vi "CTC_Test.vi"() -> ()   [LabVIEW 2011]
panel:
  out "Ain15":dbl format="%.3f"
  out "Ain14":dbl format="%.3f"
  out "Ain13":dbl format="%.3f"
  out "Ain12":dbl format="%.3f"
  out "Ain11":dbl format="%.3f"
  out "Ain10":dbl format="%.3f"
  out "Ain9":dbl format="%.3f"
  out "Ain8":dbl format="%.3f"
  out "Input err":string
  out "Din32":bool
  out "Din31":bool
  out "Din30":bool
  out "Din29":bool
  out "Din28":bool
  out "Din27":bool
  out "Din26":bool
  out "Din25":bool
  out "Din24":bool
  out "Din23":bool
  out "Din22":bool
  out "Din21":bool
  out "Din20":bool
  out "Din19":bool
  out "Din18":bool
  out "Din17":bool
  out "Din16":bool
  out "Din15":bool
  out "Din14":bool
  out "Din13":bool
  out "Din12":bool
  out "Din11":bool
  out "Din10":bool
  out "Din9":bool
  out "Din8":bool
  out "Din7":bool
  out "Din6":bool
  out "Din5":bool
  out "Din4":bool
  out "Din3":bool
  out "Din2":bool
  out "Din1":bool
  in  "Din Board":u8=1 min=1
  in  "Dout Board":u8=1 min=1
  out "Ain7":dbl format="%.3f"
  in  "Aout8":dbl min=0.0 max=2000.0 format="%.1f"
  out "Ain6":dbl format="%.3f"
  in  "Aout7":dbl min=0.0 max=2000.0 format="%.1f"
  out "Ain5":dbl format="%.3f"
  in  "Aout6":dbl min=0.0 max=2000.0 format="%.1f"
  out "Ain4":dbl format="%.3f"
  in  "Aout5":dbl min=0.0 max=2000.0 format="%.1f"
  out "Ain3":dbl format="%.3f"
  in  "Aout4":dbl min=0.0 max=2000.0 format="%.1f"
  out "Ain2":dbl format="%.3f"
  in  "Aout3":dbl min=0.0 max=2000.0 format="%.1f"
  out "Ain1":dbl format="%.3f"
  in  "Aout2":dbl min=0.0 max=2000.0 format="%.1f"
  in  "32":bool
  in  "31":bool
  in  "30":bool
  in  "29":bool
  in  "28":bool
  in  "27":bool
  in  "26":bool
  in  "25":bool
  in  "24":bool
  in  "23":bool
  in  "22":bool
  in  "21":bool
  in  "20":bool
  in  "19":bool
  in  "18":bool
  in  "17":bool
  in  "16":bool
  in  "15":bool
  in  "14":bool
  in  "13":bool
  in  "12":bool
  in  "11":bool
  in  "10":bool
  in  "9":bool
  in  "8":bool
  in  "7":bool
  in  "6":bool
  in  "5":bool
  in  "4":bool
  in  "3":bool
  in  "2":bool
  out "Ain0":dbl format="%.3f"
  in  "Aout1":dbl min=0.0 max=2000.0 format="%.1f"
  in  "1":bool
  out "set dout error":string
  in  "stop copy 2":bool
  in  "stop":bool
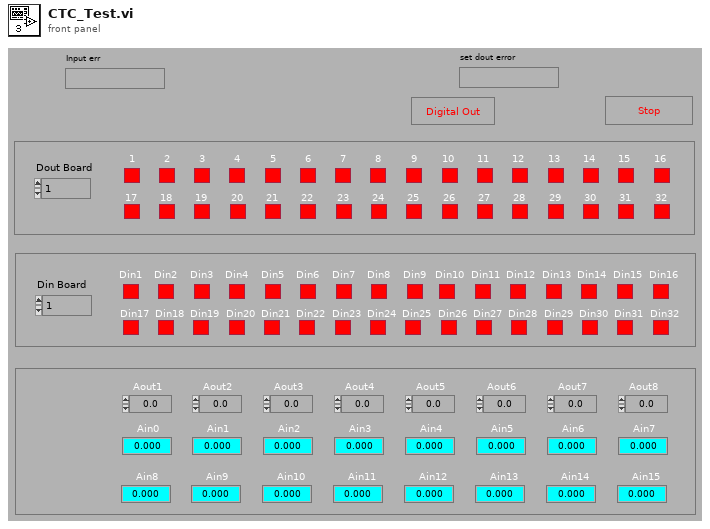
[diagram p1: front panel]
types:
  T1 = cluster{"[0]":bool, "[1]":bool, "[2]":bool, "[3]":bool, "[4]":bool, "[5]":bool, "[6]":bool, "[7]":bool, "[8]":bool, "[9]":bool, "[10]":bool, "[11]":bool, "[12]":bool, "[13]":bool, "[14]":bool, "[15]":bool}
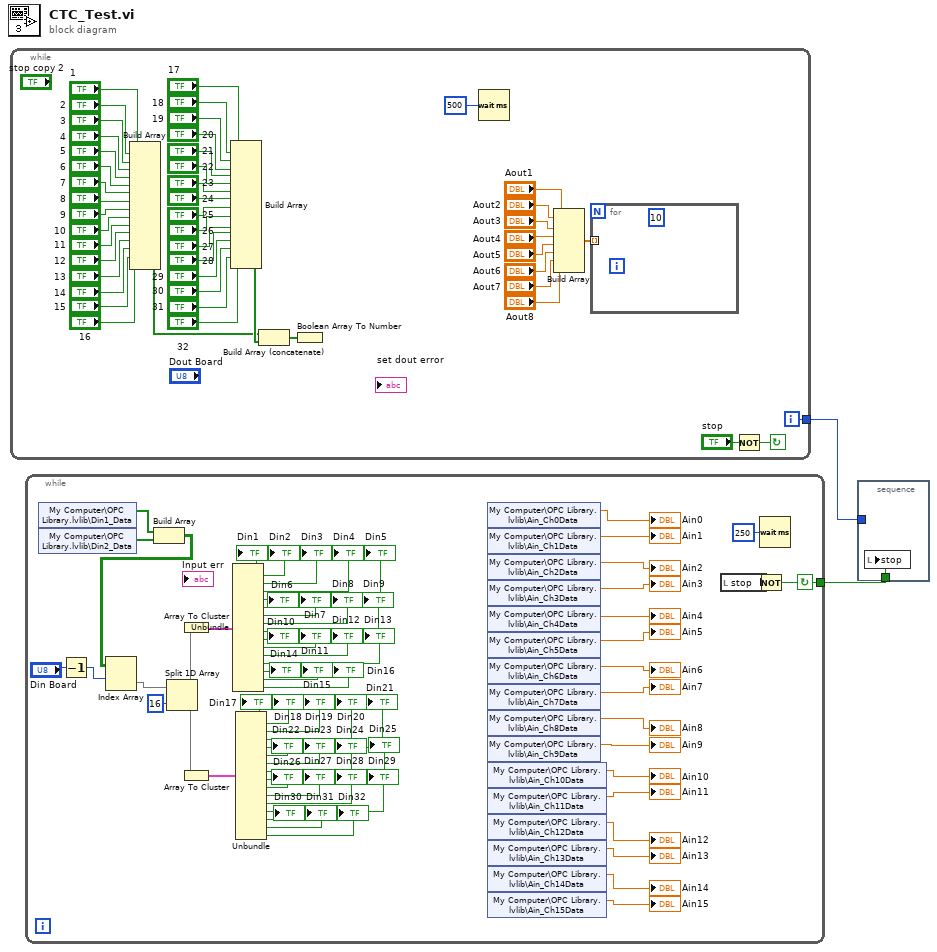
[diagram p0: block diagram]
diagram:
  n1 = while {
    tunnel: [w47] -> w2
    i -> [w47]
    stop <- w48 continue-if-true
    n2 = Build Array("1", "2", "3", "4", "5", "6", "7", "8", "9", "10", "11", "12", "13", "14", "15", "16") -> (w5:bool[])
    n3 = Build Array("17", "18", "19", "20", "21", "22", "23", "24", "25", "26", "27", "28", "29", "30", "31", "32") -> (w6:bool[])
    n4 = Build Array (concatenate)(w5, w6) -> (w4:bool[])
    n5 = Boolean Array To Number(Boolean array=w4) -> ()  [unwired: 1 out]
    n6 = Wait (ms)(milliseconds to wait=u32 500) -> ()  [unwired: 1 out]
    n7 = Build Array("Aout1", "Aout2", "Aout3", "Aout4", "Aout5", "Aout6", "Aout7", "Aout8") -> (w3:dbl[])
    n8 = for {
      tunnel: w3 -> [_] mode=indexing
      (unwired) 10
    }
    n9 = Not(x="stop") -> (.not. x?=w48:bool)
  }
  n10 = while {
    tunnel: [w111] -> w1
    stop <- w111 continue-if-true
    n11 = shared-variable "My Computer\\OPC Library.lvlib\\Din1_Data"() -> (w70:bool[])  [unwired: 1 in, 1 out]
    n12 = shared-variable "My Computer\\OPC Library.lvlib\\Din2_Data"() -> (w71:bool[])  [unwired: 1 in, 1 out]
    n13 = Decrement(x="Din Board") -> (x-1=w69:u8)
    n14 = Build Array(w70, w71) -> (w68:bool[][])
    n15 = Index Array(array=w68, index (row)=w69) -> (element=w67:bool[])  [unwired: 1 in]
    n16 = Split 1D Array(array=w67, index=16) -> (first subarray=w74:bool[], second subarray=w76:bool[])
    n17 = Array To Cluster(array=w74) -> (cluster=w75:T1)
    n18 = Array To Cluster(array=w76) -> (cluster=w77:T1)
    n19 = Unbundle(w75) -> ("[0]"=→"Din1":bool, "[1]"=→"Din2":bool, "[2]"=→"Din3":bool, "[3]"=→"Din4":bool, "[4]"=→"Din5":bool, "[5]"=→"Din6":bool, "[6]"=→"Din7":bool, "[7]"=→"Din8":bool, "[8]"=→"Din9":bool, "[9]"=→"Din10":bool, "[10]"=→"Din11":bool, "[11]"=→"Din12":bool, "[12]"=→"Din13":bool, "[13]"=→"Din14":bool, "[14]"=→"Din15":bool, "[15]"=→"Din16":bool)
    n20 = Unbundle(w77) -> ("[0]"=→"Din17":bool, "[1]"=→"Din18":bool, "[2]"=→"Din19":bool, "[3]"=→"Din20":bool, "[4]"=→"Din21":bool, "[5]"=→"Din22":bool, "[6]"=→"Din23":bool, "[7]"=→"Din24":bool, "[8]"=→"Din25":bool, "[9]"=→"Din26":bool, "[10]"=→"Din27":bool, "[11]"=→"Din28":bool, "[12]"=→"Din29":bool, "[13]"=→"Din30":bool, "[14]"=→"Din31":bool, "[15]"=→"Din32":bool)
    n21 = shared-variable "My Computer\\OPC Library.lvlib\\Ain_Ch0Data"() -> (→"Ain0":dbl)  [unwired: 1 in, 1 out]
    n22 = shared-variable "My Computer\\OPC Library.lvlib\\Ain_Ch1Data"() -> (→"Ain1":dbl)  [unwired: 1 in, 1 out]
    n23 = shared-variable "My Computer\\OPC Library.lvlib\\Ain_Ch2Data"() -> (→"Ain2":dbl)  [unwired: 1 in, 1 out]
    n24 = shared-variable "My Computer\\OPC Library.lvlib\\Ain_Ch3Data"() -> (→"Ain3":dbl)  [unwired: 1 in, 1 out]
    n25 = shared-variable "My Computer\\OPC Library.lvlib\\Ain_Ch4Data"() -> (→"Ain4":dbl)  [unwired: 1 in, 1 out]
    n26 = shared-variable "My Computer\\OPC Library.lvlib\\Ain_Ch5Data"() -> (→"Ain5":dbl)  [unwired: 1 in, 1 out]
    n27 = shared-variable "My Computer\\OPC Library.lvlib\\Ain_Ch6Data"() -> (→"Ain6":dbl)  [unwired: 1 in, 1 out]
    n28 = shared-variable "My Computer\\OPC Library.lvlib\\Ain_Ch7Data"() -> (→"Ain7":dbl)  [unwired: 1 in, 1 out]
    n29 = shared-variable "My Computer\\OPC Library.lvlib\\Ain_Ch8Data"() -> (→"Ain8":dbl)  [unwired: 1 in, 1 out]
    n30 = shared-variable "My Computer\\OPC Library.lvlib\\Ain_Ch9Data"() -> (→"Ain9":dbl)  [unwired: 1 in, 1 out]
    n31 = shared-variable "My Computer\\OPC Library.lvlib\\Ain_Ch10Data"() -> (→"Ain10":dbl)  [unwired: 1 in, 1 out]
    n32 = shared-variable "My Computer\\OPC Library.lvlib\\Ain_Ch11Data"() -> (→"Ain11":dbl)  [unwired: 1 in, 1 out]
    n33 = shared-variable "My Computer\\OPC Library.lvlib\\Ain_Ch12Data"() -> (→"Ain12":dbl)  [unwired: 1 in, 1 out]
    n34 = shared-variable "My Computer\\OPC Library.lvlib\\Ain_Ch13Data"() -> (→"Ain13":dbl)  [unwired: 1 in, 1 out]
    n35 = shared-variable "My Computer\\OPC Library.lvlib\\Ain_Ch14Data"() -> (→"Ain14":dbl)  [unwired: 1 in, 1 out]
    n36 = shared-variable "My Computer\\OPC Library.lvlib\\Ain_Ch15Data"() -> (→"Ain15":dbl)  [unwired: 1 in, 1 out]
    n37 = local read "stop"() -> (w112:bool)
    n38 = Not(x=w112) -> (.not. x?=w111:bool)
    n39 = Wait (ms)(milliseconds to wait=u32 250) -> ()  [unwired: 1 out]
  }
  n40 = stacked-sequence {
    tunnel: w2 -> [_]
    tunnel: w1 -> [w113]
    frame #0 {
      n41 = local write "stop"(w113) -> ()
    }
  }
